vi "Initialize.vi"(8 "error in":errorcluster, 11 "device data model in":refnum<class "Standard Data Model.lvclass">) -> (0 "error out":errorcluster, 3 "device data model out":refnum<class "Standard Data Model.lvclass">)   [LabVIEW 2021, in "Standard Data Model.lvclass"]
doc: "This VI initializes the device data model."
uses:
  Standard Data Model.lvclass
  Device ID Type.ctl
  Identification Parameters.ctl
  Standard Data Model.lvclass/Standard Data Model.ctl
  Device Data Model.lvclass
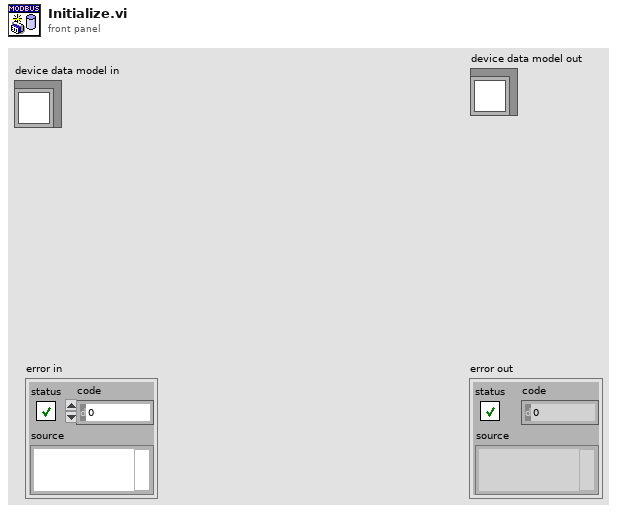
[diagram p1: front panel]
types:
  T1 = typedef "Device Data Model.lvclass/Device ID Type.ctl" = u8
  T2 = typedef "Device Data Model.lvclass/Identification Parameters.ctl" = cluster{"Object ID":u8, "Value":string}
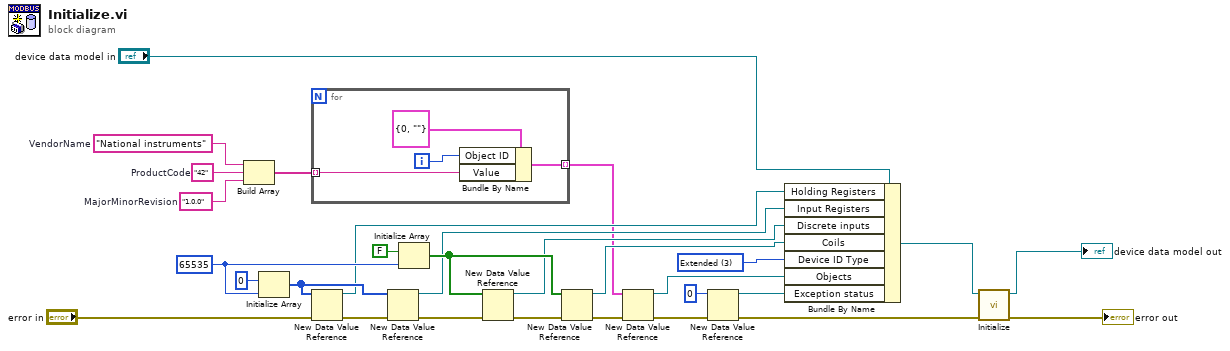
[diagram p0: block diagram]
diagram:
  w23 = T1 3 items=["Basic"=1, "Regular "=2, "Extended"=3] ("Read Device ID Code")
  w24 = "1.0.0"  # MajorMinorRevision
  w26 = "42"  # ProductCode
  w25 = "National instruments"  # VendorName
  w27 = u16 65535
  n1 = Build Array(w25, w26, w24) -> (w21:string[])
  n2 = Initialize Array(u16 0 ("Numeric"), w27) -> (w15:u16[])
  n3 = for {
    tunnel: w21 -> [w31] mode=indexing
    tunnel: [w30] -> w10 mode=indexing
    i -> [w32]
    n4 = Bundle By Name(cluster=T2 {"Object ID"=0, "Value"=""} ("Cluster"), "Object ID"=w32, "Value"=w31) -> (w30:T2)
  }
  n5 = New Data Value Reference(data value=w15, error in="error in") -> (data value reference=w11:refnum<data-value>, error out=w18:errorcluster)
  n6 = New Data Value Reference(data value=w15, error in=w18) -> (data value reference=w12:refnum<data-value>, error out=w19:errorcluster)
  n7 = Initialize Array(FALSE ("Boolean"), w27) -> (w16:bool[])
  n8 = New Data Value Reference(data value=w16, error in=w19) -> (data value reference=w13:refnum<data-value>, error out=w20:errorcluster)
  n9 = New Data Value Reference(data value=w16, error in=w20) -> (data value reference=w14:refnum<data-value>, error out=w8:errorcluster)
  n10 = New Data Value Reference(data value=w10, error in=w8) -> (data value reference=w9:refnum<data-value>, error out=w7:errorcluster)
  n11 = New Data Value Reference(data value=u8 0, error in=w7) -> (data value reference=w6:refnum<data-value>, error out=w4:errorcluster)
  n12 = Bundle By Name(cluster="device data model in", "Holding Registers"=w11, "Input Registers"=w12, "Discrete inputs"=w13, "Coils"=w14, "Device ID Type"=w23, "Objects"=w9, "Exception status"=w6) -> (w3:refnum<class "Standard Data Model.lvclass">)
  n13 = call-parent "Initialize.vi"("error in"=w4, "device data model in"=w3) -> ("error out"=→"error out":errorcluster, "device data model out"=→"device data model out":refnum<class "Standard Data Model.lvclass">)  [unwired: 8 in]
